vi "PXI Clear AO Channel Task.vi"(2 "error in":errorcluster, 3 "AO channel":string="AO01") -> (0 "error out":errorcluster)   [LabVIEW 2015]
uses:
  PXI Globals.vi
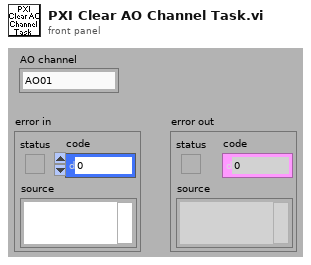
[diagram p1: front panel]
types:
  T1 = typedef "Task Struct.ctl" = cluster{"Task name":string, "Task":refnum<k21>, "Dual-channel task?":bool, "Regenerate?":bool, "Clear?":bool}
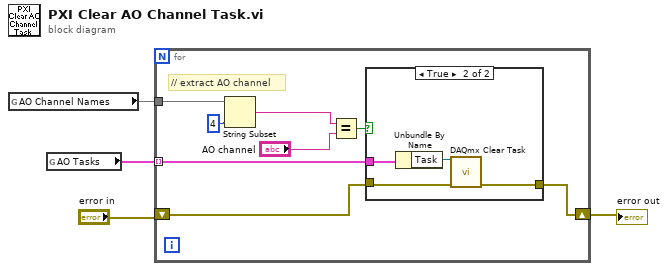
[diagram p0: block diagram]
diagram:
  n1 = global read "PXI Globals.vi" "AO Channel Names"() -> (w4)
  n2 = global read "PXI Globals.vi" "AO Tasks"() -> (w3:T1[])
  n3 = for {
    tunnel: w4 -> [w11]
    tunnel: w3 -> [w10] mode=indexing
    shift-right: [w8] -> w1
    shift-left: "error in" -> [w9]
    # "// extract AO channel"
    n4 = String Subset(string=w11, length (rest)=4 ("length (rest)")) -> (substring=w6:string)  [unwired: 1 in]
    n5 = Equal?(x=w6, y="AO channel") -> (x = y?=w7:bool)
    n6 = case shown="True" w7 {
      tunnel: w10 -> [_ w16]
      tunnel: w9 -> [w13 w15]
      tunnel: [w13 w14] -> w8
      frame False {
      }
      frame True {
        n7 = Unbundle By Name(w16) -> ("Task"=w17:refnum<k21>)
        n8 = call <vilib>:"DAQmx Clear Task.vi"("task in"=w17, "error in"=w15) -> ("error out"=w14:errorcluster)  [unwired: 13 in]
      }
    }
  }
  "error out" <- w1
